vi "CreateFactory.vi"(6 "Agent Class Path":path, 7 "Library Base Path":path, 8 "error in":errorcluster, 10 "Visitor Class Paths":path[](array[path]), 11 "Class Name":string) -> (0 "error out":errorcluster, 2 "Created Classes":path[](array[path]))   [LabVIEW 2009, in "HGF_VisitorGenerator.lvlib"]
doc: "create factory class and override classes.vi containing default objects of agent and visitor classes"
uses:
  HGF_VisitorGenerator.lvlib
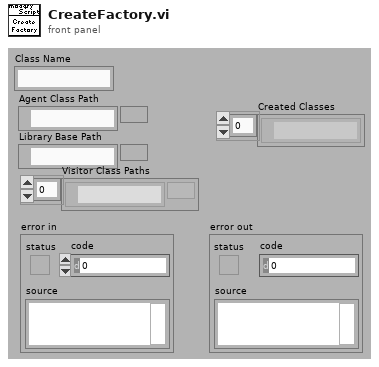
[diagram p1: front panel]
types:
  T1 = enum32{"invalid scope", "public", "private", "protected", "community"}
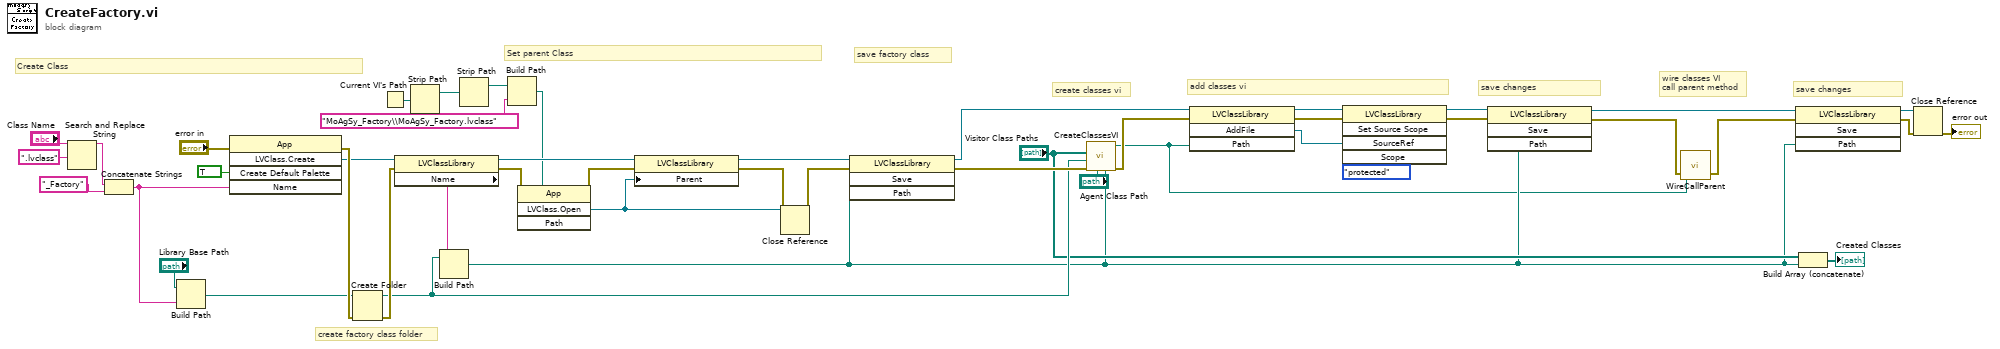
[diagram p0: block diagram]
diagram:
  # "wire classes VI\ncall parent method"
  # "save changes"
  # "save changes"
  # "add classes vi"
  # "create classes vi"
  # "create factory class folder"
  # "save factory class"
  # "Set parent Class"
  # "Create Class"
  n1 = Search and Replace String(input string="Class Name", search string=".lvclass") -> (result string=w22:string)  [unwired: 6 in, 3 out]
  n2 = Concatenate Strings(w22, "_Factory" ("string")) -> (w26:string)
  n3 = Build Path(base path="Library Base Path", name or relative path=w26) -> (appended path=w30:path)
  n4 = invoke class="App" method="LVClass.Create"(error in="error in", "Create Default Palette"=TRUE ("Create:Default Palette"), "Name"=w26) -> (error out=w32:errorcluster, "LVClass.Create"=w28:refnum<vi>)  [unwired: 2 in, 3 out]
  n5 = Create Folder(path (use dialog)=w30, error in=w32) -> (created path=w15:path, error out=w36:errorcluster)  [unwired: 1 in, 1 out]
  n6 = Current VI's Path() -> (path=w5:path)
  n7 = property class="LVClassLibrary"(reference=w28, error in=w36) -> (reference out=w35:refnum<vi>, error out=w34:errorcluster, "Name"=w29:string)
  n8 = Strip Path(path=w5) -> (stripped path=w4:path)  [unwired: 1 out]
  n9 = Build Path(base path=w15, name or relative path=w29) -> (appended path=w9:path)
  n10 = Strip Path(path=w4) -> (stripped path=w3:path)  [unwired: 1 out]
  n11 = Build Path(base path=w3, name or relative path="MoAgSy_Factory\\MoAgSy_Factory.lvclass") -> (appended path=w1:path)
  n12 = invoke class="App" method="LVClass.Open"(error in=w34, "Path"=w1) -> (error out=w33:errorcluster, "LVClass.Open"=w37:refnum<vi>)  [unwired: 2 in, 2 out]
  n13 = property class="LVClassLibrary"(reference=w35, error in=w33, "Parent"=w37) -> (reference out=w40:refnum<vi>, error out=w38:errorcluster)
  n14 = Close Reference(reference=w37, error in (no error)=w38) -> (error out=w39:errorcluster)
  n15 = invoke class="LVClassLibrary" method="Save"(reference=w40, error in=w39, "Path"=w9) -> (reference out=w31:refnum<vi>, error out=w17:errorcluster)  [unwired: 1 in, 2 out]
  n16 = call "CreateClassesVI.vi"("Factory Class Path"=w9, "Agents class path"="Agent Class Path", "error in"=w17, "FactoryFolder"=w15, "Visitor Class Paths"="Visitor Class Paths") -> ("error out"=w18:errorcluster, "classesVIPath"=w6:path)  [unwired: 5 in]
  n17 = invoke class="LVClassLibrary" method="AddFile"(reference=w31, error in=w18, "Path"=w6) -> (reference out=w41:refnum<vi>, error out=w43:errorcluster, "AddFile"=w45:refnum<vi>)  [unwired: 1 in, 1 out]
  n18 = invoke class="LVClassLibrary" method="Set Source Scope"(reference=w41, error in=w43, "SourceRef"=w45, "Scope"=T1."protected" ("scope")) -> (reference out=w42:refnum<vi>, error out=w46:errorcluster)  [unwired: 1 in, 3 out]
  n19 = invoke class="LVClassLibrary" method="Save"(reference=w42, error in=w46, "Path"=w9) -> (reference out=w12:refnum<vi>, error out=w8:errorcluster)  [unwired: 1 in, 2 out]
  n20 = call "WireCallParent.vi"("error in (no error)"=w8, "classesVIPath"=w6) -> ("error out"=w7:errorcluster)  [unwired: 1 in]
  n21 = invoke class="LVClassLibrary" method="Save"(reference=w12, error in=w7, "Path"=w9) -> (reference out=w11:refnum<vi>, error out=w10:errorcluster)  [unwired: 1 in, 2 out]
  n22 = Build Array (concatenate)("Visitor Class Paths", w9) -> (→"Created Classes":path[])
  n23 = Close Reference(reference=w11, error in (no error)=w10) -> (error out=→"error out":errorcluster)
